vi "TestCode.vi"() -> ()   [LabVIEW 2020]
panel:
  out "a 2":dbl[](array[numeric])
  out "a":dbl[](array[numeric])
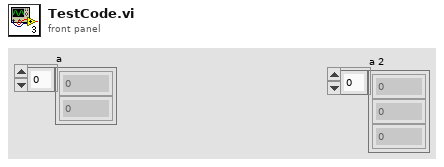
[diagram p1: front panel]
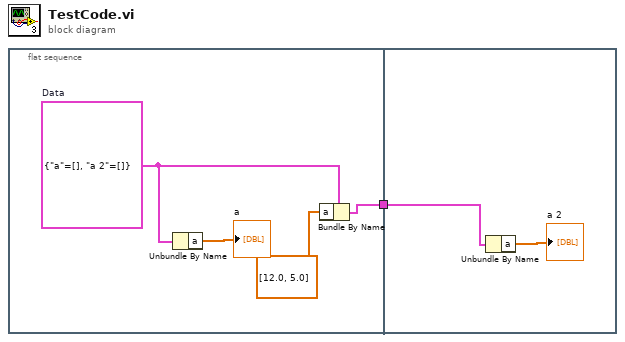
[diagram p0: block diagram]
diagram:
  n1 = flat-sequence {
    tunnel: [w2] -> w1
    tunnel: w1 -> [w6]
    frame #0 {
      w4 = cluster{"a":dbl[], "a 2":dbl[]} {"a"=[], "a 2"=[]}  # Data
      n2 = Unbundle By Name(w4) -> ("a"=→"a":dbl[])
      n3 = Bundle By Name(cluster=w4, "a"=dbl[] [12.0, 5.0]) -> (w2:cluster{"a":dbl[], "a 2":dbl[]})
    }
    frame #1 {
      n4 = Unbundle By Name(w6) -> ("a"=→"a 2":dbl[])
    }
  }
